vi "Vision Processing.vi"(4 "error in (no error)":errorcluster) -> ()   [LabVIEW 2013]
doc: "This VI runs in parallel to other tasks. It gets images from the camera, processes them for color or shape and use that information to affect robot behavior."
uses:
  Robot Global Data.vi
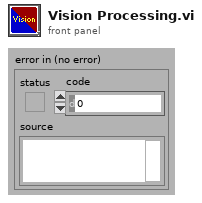
[diagram p1: front panel]
types:
  T1 = typedef "Image Type" = u32
  T2 = typedef "WPI_CameraDevRef.ctl" = cluster{"Camera Address":string, "CameraStatus":errorcluster, "Acquire Image Notifier":refnum<notifier>}
  T3 = typedef "IMAQ Image.ctl" = refnum<image>
  T4 = typedef "WPI_CameraImageSize.ctl" = enum16{"640x480", "320x240", "160x120"}
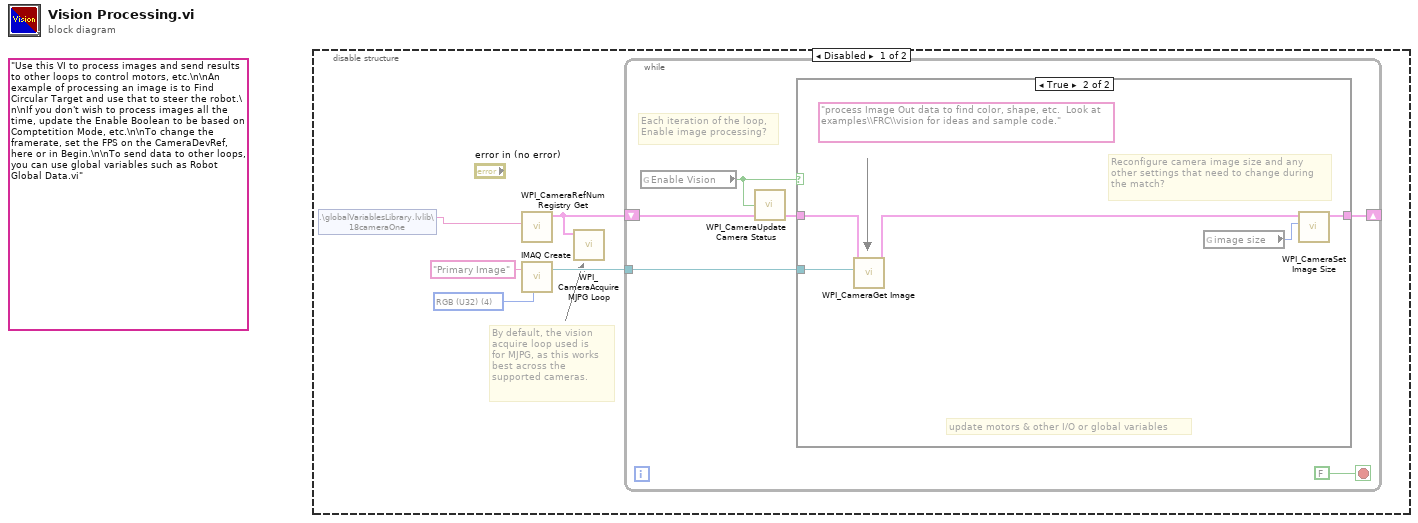
[diagram p0: block diagram]
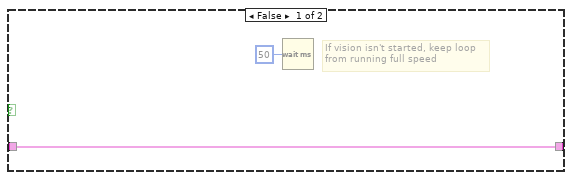
[diagram p2: hidden frame]
diagram:
  (unwired) "Use this VI to process images and send results to other loops to control motors, etc.\n\nAn example of processing an image is to Find Circular Target and use that to steer the robot.\n\nIf you don't wish to process images all the time, update the Enable Boolean to be based on Comptetition Mode, etc.\n\nTo change the framerate, set the FPS on the CameraDevRef, here or in Begin.\n\nTo send data to other loops, you can use global variables such as Robot Global Data.vi"
  n1 = disable-structure shown="Disabled" {
    frame Disabled {
      w5 = T1 4 items=["Grayscale (U8)", "Grayscale (I16)", "Grayscale (SGL)", "Complex (CSG)", "RGB (U32)", "HSL (U32)", "RGB (U64)"] ("Image Type")
      # "By default, the vision\nacquire loop used is\nfor MJPG, as this works\nbest across the\nsupported cameras."
      n2 = shared-variable ".\\globalVariablesLibrary.lvlib\\18cameraOne"() -> (w1:string)  [unwired: 1 in, 1 out]
      n3 = call <vilib>:"WPI_CameraRefNum Registry Get.vi"("refnum name"=w1) -> ("CameraDevRef"=w2:T2)  [unwired: 1 in, 9 out]
      n4 = call "IMAQ Create"("Image Name"="Primary Image", "Image Type"=w5) -> ("New Image"=w3:T3)  [unwired: 2 in, 2 out]
      n5 = call <vilib>:"WPI_CameraAcquire MJPG Loop.vi"("CameraDevRef"=w2) -> ()  [unwired: 11 in]
      n6 = while {
        shift-right: [w10] -> _
        shift-left: w2 -> [w8]
        tunnel: w3 -> [w9]
        stop <- FALSE stop-if-true
        # "Each iteration of the loop,\nEnable image processing?"
        n7 = global read "Robot Global Data.vi" "Enable Vision"() -> (w6:bool)
        n8 = call <vilib>:"WPI_CameraUpdate Camera Status.vi"("CameraDevRef In"=w8, "Enable Vision"=w6) -> ("CameraDevRef Out"=w7:T2)  [unwired: 3 in]
        n9 = case shown="True" w6 {
          tunnel: w9 -> [_ w17]
          tunnel: [w13 w18] -> w10
          tunnel: w7 -> [w13 w15]
          frame False {
            # "If vision isn't started, keep loop\nfrom running full speed"
            n10 = Wait (ms)(milliseconds to wait=u32 50) -> ()  [unwired: 1 out]
          }
          frame True {
            (unwired) "process Image Out data to find color, shape, etc.  Look at examples\\FRC\\vision for ideas and sample code."
            # "update motors & other I/O or global variables"
            # "Reconfigure camera image size and any\nother settings that need to change during\nthe match?"
            n11 = call <vilib>:"WPI_CameraGet Image.vi"("Image"=w17, "CameraDevRef"=w15) -> ("CameraDevRef Out"=w14:T2)  [unwired: 1 in, 8 out]
            n12 = global read "Robot Global Data.vi" "image size"() -> (w16:T4)
            n13 = call <vilib>:"WPI_CameraSet Image Size.vi"("Image Size"=w16, "CameraDevRef"=w14) -> ("CameraDevRef Out"=w18:T2)  [unwired: 1 in, 8 out]
          }
        }
      }
    }
    frame Enabled {
    }
  }
